vi "ReadMaxAmp.vi"(8 "error in (no error)":errorcluster, 9 "Channel":dbl=1.0, 11 "Tek 2k in":refnum<class "Tek 2k Scope.lvclass">) -> (0 "error out":errorcluster, 1 "Amplitude":dbl, 3 "Tek 2k out":refnum<class "Tek 2k Scope.lvclass">)   [LabVIEW 2010, in "Tek 2k Scope.lvclass"]
uses:
  Tek 2k Scope.lvclass
  Tek 2k Scope.lvclass/Tek 2k Scope.ctl
  <instrlib>/Tektronix TDS 200 1000 2000 Series/Tektronix TDS 200 1000 2000 Series.lvlib
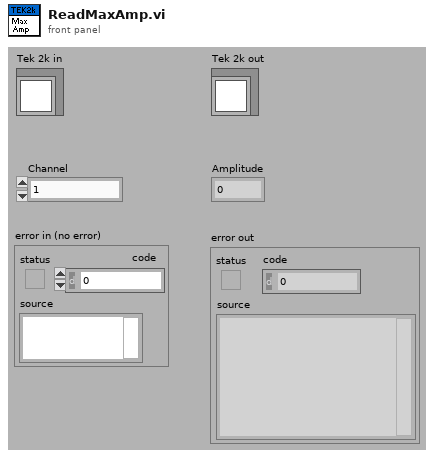
[diagram p1: front panel]
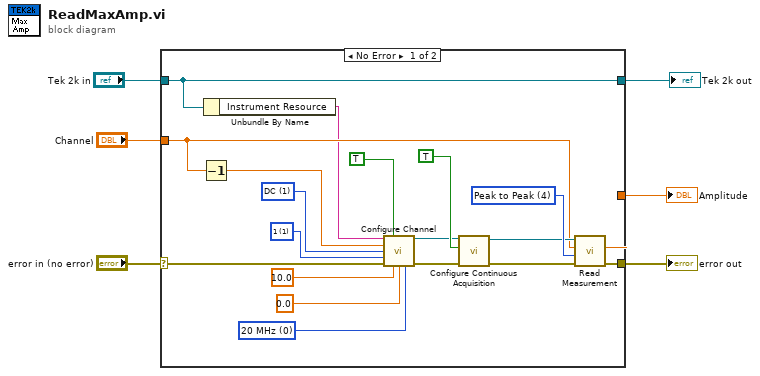
[diagram p0: block diagram]
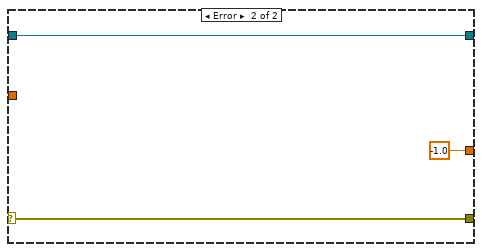
[diagram p2: hidden frame]
diagram:
  n1 = case shown="No Error" "error in (no error)" {
    selector: "error in (no error)" -> [w9 w28]
    tunnel: [w14 w28] -> w5
    tunnel: "Channel" -> [w11 _]
    tunnel: [w18 -1.0] -> w4
    tunnel: "Tek 2k in" -> [w8 w26]
    tunnel: [w8 w26] -> w2
    frame No Error {
      w19 = u16 4 items=["Frequency", "Mean", "Period", "Phase", "Peak to Peak", "Complete RMS", "Minimum", "Maximum", "Rise Time", "Fall Time", "Positive Width", "Negative Width"] ("Measurement Type (0: Frequency)")
      w24 = u16 1 items=["AC", "DC", "Ground"] ("Vertical Coupling (1: DC)")
      w20 = 0 items=["20 MHz", "Unlimited"] ("Bandwidth (0: 20 MHz)")
      w23 = 1 items=["1"=1, "10"=10, "20"=20, "50"=50, "100"=100, "500"=500, "1000"=1000] ("Probe Attenuation (10: 10X)")
      n2 = Decrement(x=w11) -> (x-1=w10:dbl)
      n3 = Unbundle By Name(w8) -> ("Instrument Resource"=w7:string)
      n4 = call <instrlib>:"Configure Channel.vi"("VISA resource name"=w7, "Enable Channel (True)"=TRUE, "Channel (0: Channel 1)"=w10, "Vertical Coupling (1: DC)"=w24, "Probe Attenuation (10: 10X)"=w23, "error in (no error)"=w9, "Vertical Range (10.0 V/div)"=10.0 ("Vertical Range (10.0 V)"), "Vertical Offset (0.0 divs)"=0.0, "Bandwidth (0: 20 MHz)"=w20) -> ("VISA resource name out"=w16:refnum<visa-resource-name>, "error out"=w15:errorcluster)  [unwired: 5 out]
      n5 = call <instrlib>:"Configure Continuous Acquisition.vi"("error in (no error)"=w15, "Enable Continuous Acquisition Mode (True)"=TRUE, "VISA resource name"=w16) -> ("error out"=w12:errorcluster, "VISA resource name out"=w13:refnum<visa-resource-name>)  [unwired: 7 out]
      n6 = call <instrlib>:"Read Measurement.vi"("error in (no error)"=w12, "Measurement Type (0: Frequency)"=w19, "Channel (1: Channel 1)"=w11, "VISA resource name"=w13) -> ("error out"=w14:errorcluster, "Measurement"=w18:dbl)  [unwired: 6 out]
    }
    frame Error {
    }
  }
  "error out" <- w5
  "Amplitude" <- w4
  "Tek 2k out" <- w2
